vi "Buffer Current Data.vi"(8 "error in (no error)":errorcluster, 11 "Model in":refnum<class "Model.lvclass">) -> (0 "error out":errorcluster, 3 "Model out":refnum<class "Model.lvclass">)   [LabVIEW 2016, in "Model.lvclass"]
uses:
  Model.lvclass
  Model.lvclass/Model.ctl
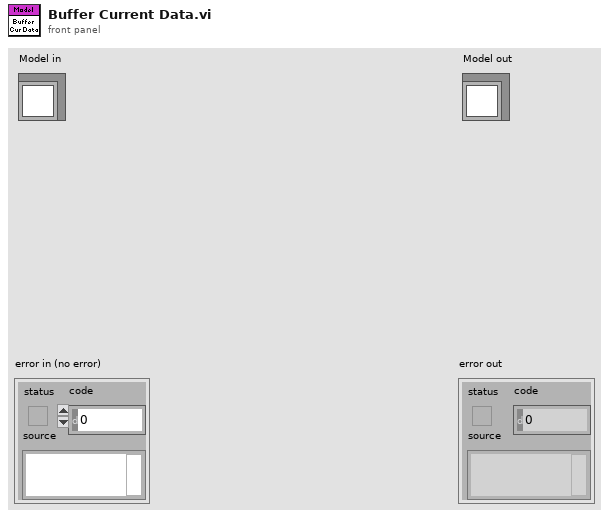
[diagram p1: front panel]
types:
  T1 = typedef "HPMT_Typedefs.lvlib/ActuatorData.ctl" = cluster{"Timestamp":dbl, "Force":dbl, "Encoder Value":i32, "Displacement Sensor 1":dbl, "Displacement Sensor 2":dbl, "Limit Switch CW":bool, "Limit Switch CCW":bool}
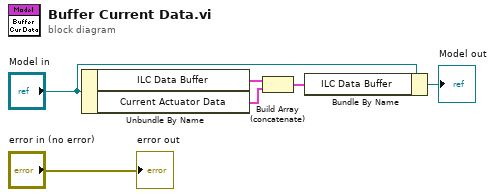
[diagram p0: block diagram]
diagram:
  n1 = Unbundle By Name("Model in") -> ("ILC Data Buffer"=w6:T1[], "Current Actuator Data"=w5:T1)
  n2 = Build Array (concatenate)(w6, w5) -> (w2:T1[])
  n3 = Bundle By Name(cluster="Model in", "ILC Data Buffer"=w2) -> (→"Model out":refnum<class "Model.lvclass">)
  "error out" <- "error in (no error)"
